vi "Write Data.vi"(8 "error in (no error)":errorcluster, 9 "Publication Time":timestamp, 10 "Value":variant, 11 "StreamToDiskTransport In":refnum<class "StreamToDiskTransport.lvclass">) -> (0 "error out":errorcluster, 3 "StreamToDiskTransport Out":refnum<class "StreamToDiskTransport.lvclass">)   [LabVIEW 2015, in "Transport.lvlib" / "StreamToDiskTransport.lvclass"]
doc: "<License>\nCopyright © 2017 Composed Systems, LLC | All rights reserved\nwww.composed.io\n\nAuthor: Ethan Stern <ethan.stern@composed.io>\n\nThis software is provided \"AS IS\" WITHOUT WARRANTIES, either express or implied, AND IS FOR EDUCATIONAL PURPOSES ONLY.\n</License>"
uses:
  StreamToDiskTransport.lvclass
  StreamToDiskTransport.lvclass/StreamToDiskTransport.ctl
  <vilib>/Utility/error.llb/Error Cluster From Error Code.vi
  <vilib>/ErrorRing/Error Ring.xnode
  <vilib>/Utility/Data Type/NI_Data Type.lvlib
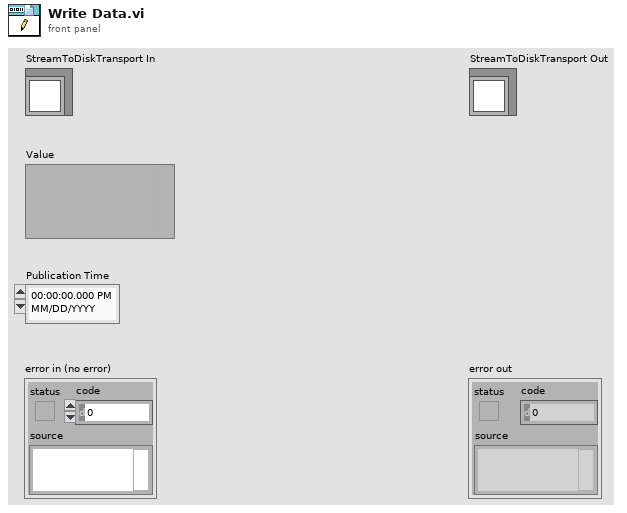
[diagram p1: front panel]
types:
  T1 = typedef "NI_Data Type.lvlib/Data Type.ctl" = enum8{"Invalid Type", "Void", "I8", "I16", "I32", "I64", "U8", "U16", "U32", "U64", "Single Float", "Double Float", "Extended Float", "Single Complex", "Double Complex", "Extended Complex", "Enum U8", "Enum U16", "Enum U32", "Enum U64", "Single Float With Unit", "Double Float With Unit", "Extended Float With Unit", "Single Complex with Unit", "Double Complex with Unit", "Extended Complex with Unit", "Boolean", "String", "Path", "Picture", "Tag", "Array", "Cluster", "Variant", "LV Variant", "Waveform", "Timestamp", "Digital Waveform", "Digital Data", "ExpressData", "Refnum", "External Data", "VI", "Poly VI", "LabVIEW Class Instance", "Fixed Point"}
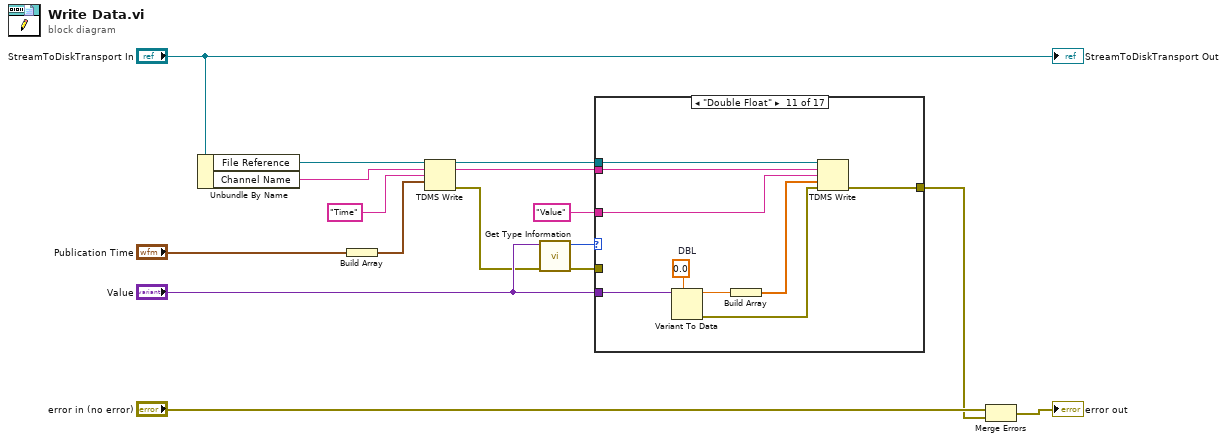
[diagram p0: block diagram]
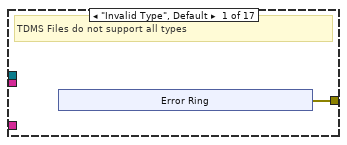
[diagram p2: hidden frame]
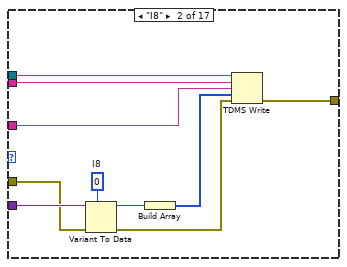
[diagram p3: hidden frame]
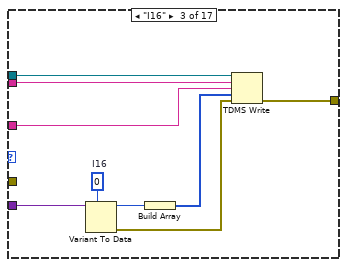
[diagram p4: hidden frame]
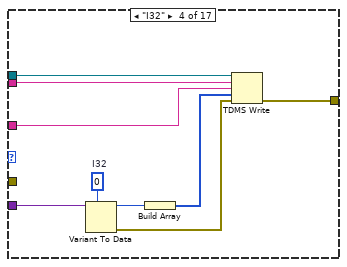
[diagram p5: hidden frame]
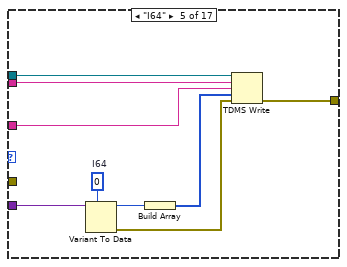
[diagram p6: hidden frame]
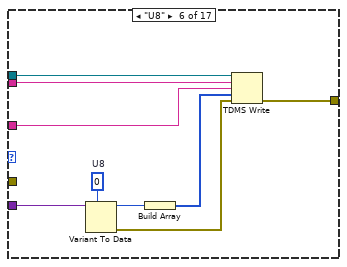
[diagram p7: hidden frame]
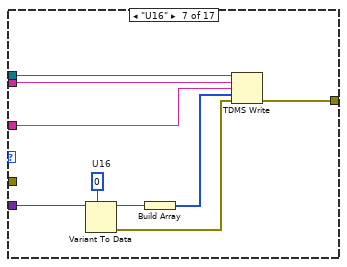
[diagram p8: hidden frame]
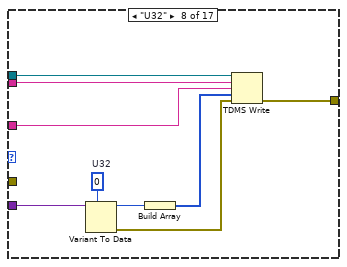
[diagram p9: hidden frame]
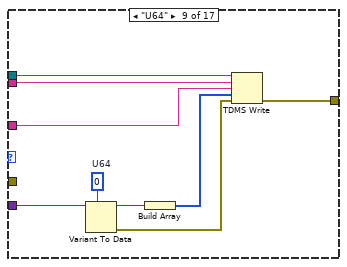
[diagram p10: hidden frame]
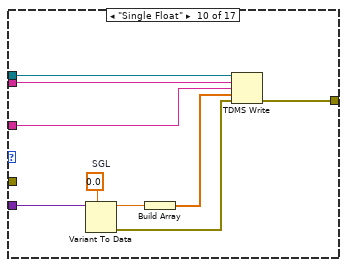
[diagram p11: hidden frame]
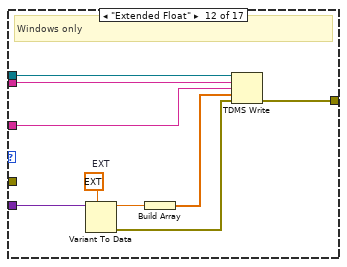
[diagram p12: hidden frame]
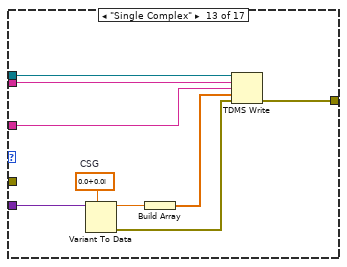
[diagram p13: hidden frame]
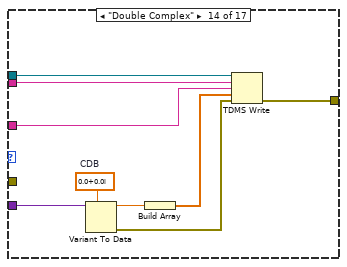
[diagram p14: hidden frame]
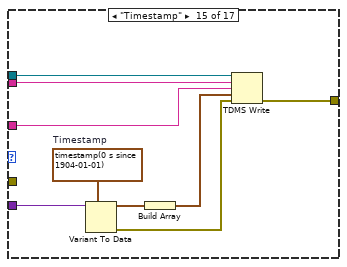
[diagram p15: hidden frame]
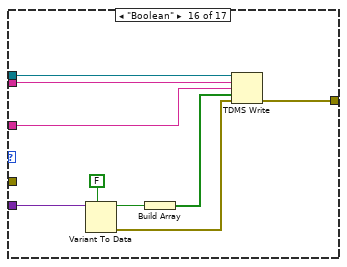
[diagram p16: hidden frame]
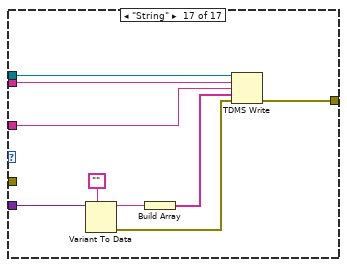
[diagram p17: hidden frame]
diagram:
  n1 = Unbundle By Name("StreamToDiskTransport In") -> ("File Reference"=w8:refnum<k34>, "Channel Name"=w7:string)
  n2 = Build Array("Publication Time") -> (w3:timestamp[])
  n3 = TDMS Write(0:w8, 5:w7, 7:"Time" ("channel name(s) in (Untitled)"), 9:w3) -> (4:w5:refnum<k34>, 6:w6:string, 15:w2:errorcluster)  [unwired: 2 in, 1 out]
  n4 = call <vilib>:"Get Type Information.vi"("error in (no error)"=w2, "Variant"="Value") -> ("error out"=w1:errorcluster, "Type"=w10:T1)  [unwired: 5 in, 3 out]
  n5 = case shown="\"Double Float\"" w10 {
    tunnel: [w17 w31 w40 w49 w58 w67 w76 w85 w94 w103 w112 w121 w130 w139 w148 w157 w166] -> w13
    tunnel: w6 -> [_ w25 w34 w43 w52 w61 w70 w79 w88 w97 w106 w115 w124 w133 w142 w151 w160]
    tunnel: "Value" -> [_ w24 w33 w42 w51 w60 w69 w78 w87 w96 w105 w114 w123 w132 w141 w150 w159]
    tunnel: w5 -> [_ w26 w35 w44 w53 w62 w71 w80 w89 w98 w107 w116 w125 w134 w143 w152 w161]
    tunnel: "Value" ("channel name(s) in (Untitled)") -> [_ w28 w37 w46 w55 w64 w73 w82 w91 w100 w109 w118 w127 w136 w145 w154 w163]
    tunnel: w1 -> [_ w22 _ _ _ _ _ _ _ _ _ _ _ _ _ _ _]
    frame "Invalid Type", Default {
      # "TDMS Files do not support all types"
      n6 = xnode "Error Ring"() -> ("error out"=w17:errorcluster)
    }
    frame "I8" {
      w29 = i8 0  # I8
      n7 = Variant To Data(error in=w22, type=w29, Variant=w24) -> (data=w23:i8, error out=w27:errorcluster)
      n8 = Build Array(w23) -> (w30:i8[])
      n9 = TDMS Write(0:w26, 5:w25, 7:w28, 9:w30, 11:w27) -> (15:w31:errorcluster)  [unwired: 1 in, 3 out]
    }
    frame "I16" {
      w38 = i16 0  # I16
      n10 = Variant To Data(type=w38, Variant=w33) -> (data=w32:i16, error out=w36:errorcluster)  [unwired: 1 in]
      n11 = Build Array(w32) -> (w39:i16[])
      n12 = TDMS Write(0:w35, 5:w34, 7:w37, 9:w39, 11:w36) -> (15:w40:errorcluster)  [unwired: 1 in, 3 out]
    }
    frame "I32" {
      w47 = 0  # I32
      n13 = Variant To Data(type=w47, Variant=w42) -> (data=w41:i32, error out=w45:errorcluster)  [unwired: 1 in]
      n14 = Build Array(w41) -> (w48:i32[])
      n15 = TDMS Write(0:w44, 5:w43, 7:w46, 9:w48, 11:w45) -> (15:w49:errorcluster)  [unwired: 1 in, 3 out]
    }
    frame "I64" {
      w56 = i64 0  # I64
      n16 = Variant To Data(type=w56, Variant=w51) -> (data=w50:i64, error out=w54:errorcluster)  [unwired: 1 in]
      n17 = Build Array(w50) -> (w57:i64[])
      n18 = TDMS Write(0:w53, 5:w52, 7:w55, 9:w57, 11:w54) -> (15:w58:errorcluster)  [unwired: 1 in, 3 out]
    }
    frame "U8" {
      w65 = u8 0  # U8
      n19 = Variant To Data(type=w65, Variant=w60) -> (data=w59:u8, error out=w63:errorcluster)  [unwired: 1 in]
      n20 = Build Array(w59) -> (w66:u8[])
      n21 = TDMS Write(0:w62, 5:w61, 7:w64, 9:w66, 11:w63) -> (15:w67:errorcluster)  [unwired: 1 in, 3 out]
    }
    frame "U16" {
      w74 = u16 0  # U16
      n22 = Variant To Data(type=w74, Variant=w69) -> (data=w68:u16, error out=w72:errorcluster)  [unwired: 1 in]
      n23 = Build Array(w68) -> (w75:u16[])
      n24 = TDMS Write(0:w71, 5:w70, 7:w73, 9:w75, 11:w72) -> (15:w76:errorcluster)  [unwired: 1 in, 3 out]
    }
    frame "U32" {
      w83 = u32 0  # U32
      n25 = Variant To Data(type=w83, Variant=w78) -> (data=w77:u32, error out=w81:errorcluster)  [unwired: 1 in]
      n26 = Build Array(w77) -> (w84:u32[])
      n27 = TDMS Write(0:w80, 5:w79, 7:w82, 9:w84, 11:w81) -> (15:w85:errorcluster)  [unwired: 1 in, 3 out]
    }
    frame "U64" {
      w92 = u64 0  # U64
      n28 = Variant To Data(type=w92, Variant=w87) -> (data=w86:u64, error out=w90:errorcluster)  [unwired: 1 in]
      n29 = Build Array(w86) -> (w93:u64[])
      n30 = TDMS Write(0:w89, 5:w88, 7:w91, 9:w93, 11:w90) -> (15:w94:errorcluster)  [unwired: 1 in, 3 out]
    }
    frame "Single Float" {
      w101 = sgl 0.0  # SGL
      n31 = Variant To Data(type=w101, Variant=w96) -> (data=w95:sgl, error out=w99:errorcluster)  [unwired: 1 in]
      n32 = Build Array(w95) -> (w102:sgl[])
      n33 = TDMS Write(0:w98, 5:w97, 7:w100, 9:w102, 11:w99) -> (15:w103:errorcluster)  [unwired: 1 in, 3 out]
    }
    frame "Double Float" {
      w110 = 0.0  # DBL
      n34 = Variant To Data(type=w110, Variant=w105) -> (data=w104:dbl, error out=w108:errorcluster)  [unwired: 1 in]
      n35 = Build Array(w104) -> (w111:dbl[])
      n36 = TDMS Write(0:w107, 5:w106, 7:w109, 9:w111, 11:w108) -> (15:w112:errorcluster)  [unwired: 1 in, 3 out]
    }
    frame "Extended Float" {
      w119 = ext 0.0  # EXT
      # "Windows only"
      n37 = Variant To Data(type=w119, Variant=w114) -> (data=w113:ext, error out=w117:errorcluster)  [unwired: 1 in]
      n38 = Build Array(w113) -> (w120:ext[])
      n39 = TDMS Write(0:w116, 5:w115, 7:w118, 9:w120, 11:w117) -> (15:w121:errorcluster)  [unwired: 1 in, 3 out]
    }
    frame "Single Complex" {
      w128 = csg 0.0+0.0i  # CSG
      n40 = Variant To Data(type=w128, Variant=w123) -> (data=w122:csg, error out=w126:errorcluster)  [unwired: 1 in]
      n41 = Build Array(w122) -> (w129:csg[])
      n42 = TDMS Write(0:w125, 5:w124, 7:w127, 9:w129, 11:w126) -> (15:w130:errorcluster)  [unwired: 1 in, 3 out]
    }
    frame "Double Complex" {
      w137 = cdb 0.0+0.0i  # CDB
      n43 = Variant To Data(type=w137, Variant=w132) -> (data=w131:cdb, error out=w135:errorcluster)  [unwired: 1 in]
      n44 = Build Array(w131) -> (w138:cdb[])
      n45 = TDMS Write(0:w134, 5:w133, 7:w136, 9:w138, 11:w135) -> (15:w139:errorcluster)  [unwired: 1 in, 3 out]
    }
    frame "Timestamp" {
      w146 = timestamp(0 s since 1904-01-01)  # Timestamp
      n46 = Variant To Data(type=w146, Variant=w141) -> (data=w140:timestamp, error out=w144:errorcluster)  [unwired: 1 in]
      n47 = Build Array(w140) -> (w147:timestamp[])
      n48 = TDMS Write(0:w143, 5:w142, 7:w145, 9:w147, 11:w144) -> (15:w148:errorcluster)  [unwired: 1 in, 3 out]
    }
    frame "Boolean" {
      n49 = Variant To Data(type=FALSE, Variant=w150) -> (data=w149:bool, error out=w153:errorcluster)  [unwired: 1 in]
      n50 = Build Array(w149) -> (w156:bool[])
      n51 = TDMS Write(0:w152, 5:w151, 7:w154, 9:w156, 11:w153) -> (15:w157:errorcluster)  [unwired: 1 in, 3 out]
    }
    frame "String" {
      n52 = Variant To Data(type="", Variant=w159) -> (data=w158:string, error out=w162:errorcluster)  [unwired: 1 in]
      n53 = Build Array(w158) -> (w165:string[])
      n54 = TDMS Write(0:w161, 5:w160, 7:w163, 9:w165, 11:w162) -> (15:w166:errorcluster)  [unwired: 1 in, 3 out]
    }
  }
  n55 = Merge Errors("error in (no error)", w13) -> (→"error out":errorcluster)
  "StreamToDiskTransport Out" <- "StreamToDiskTransport In"
